vi "WM Low Pass Filter.vi"(1 "Cutoff Freq":dbl format="%.2f", 2 "Sampling Freq":dbl format="%.2f", 3 "Input":dbl[](array[numeric]) format="%.2f") -> (0 "Output":dbl[](array[numeric]) format="%.2f")   [LabVIEW 2012]
uses:
  <vilib>/Analysis/2dsp.llb/Real FFT.vi
  <vilib>/Analysis/2dsp.llb/Inverse Real FFT.vi
  <vilib>/Analysis/NI_AALPro.lvlib
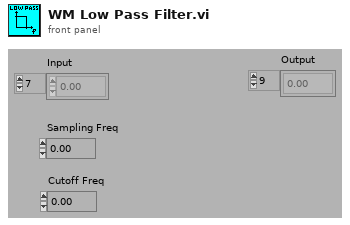
[diagram p1: front panel]
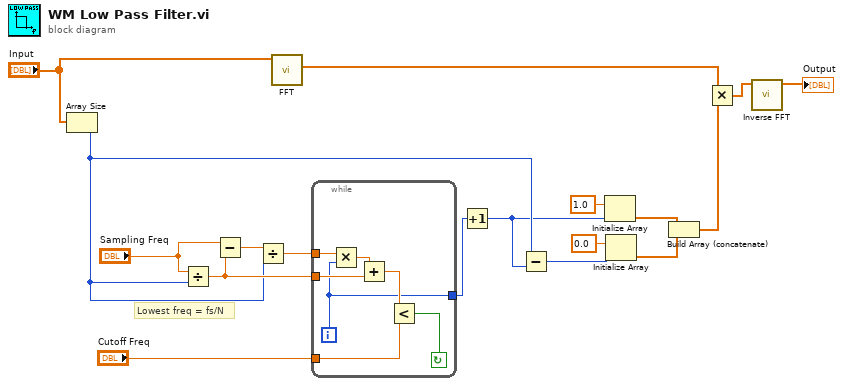
[diagram p0: block diagram]
diagram:
  # "Lowest freq = fs/N"
  n1 = Array Size(array="Input") -> (size(s)=w3:i32)
  n2 = Divide(x="Sampling Freq", y=w3) -> (x/y=w8:dbl)
  n3 = Subtract(x="Sampling Freq", y=w8) -> (x-y=w9:dbl)
  n4 = Divide(x=w9, y=w3) -> (x/y=w7:dbl)
  n5 = call-poly <vilib>:"FFT.vi"("X"="Input") -> ("FFT {X}"=w18:cdb[])  [unwired: 9 in, 1 out]
  n6 = while {
    tunnel: [w19] -> w5
    tunnel: "Cutoff Freq" -> [w21]
    tunnel: w7 -> [w24]
    tunnel: w8 -> [w25]
    i -> [w19]
    stop <- w20 continue-if-true
    n7 = Multiply(x=w24, y=w19) -> (x*y=w23:dbl)
    n8 = Add(x=w23, y=w25) -> (x+y=w22:dbl)
    n9 = Less?(x=w22, y=w21) -> (x < y?=w20:bool)
  }
  n10 = Increment(x=w5) -> (x+1=w2:i32)
  n11 = Subtract(x=w3, y=w2) -> (x-y=w4:i32)
  n12 = Initialize Array(1.0 ("Element Data"), w2) -> (w12:dbl[])
  n13 = Initialize Array(0.0 ("Element Data"), w4) -> (w11:dbl[])
  n14 = Build Array (concatenate)(w12, w11) -> (w10:dbl[])
  n15 = Multiply(x=w18, y=w10) -> (x*y=w17:cdb[])
  n16 = call-poly <vilib>:"Inverse FFT.vi"("FFT {X}"=w17) -> ("X"=→"Output":dbl[])  [unwired: 9 in, 1 out]
